vi "String to Array.vi"(0 "string":string, 1 "delimiter (;)":string=";") -> (2 "array":string[](array[string]))   [LabVIEW 2017]
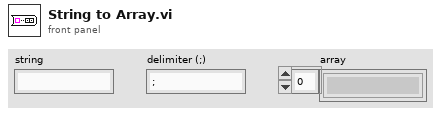
[diagram p1: front panel]
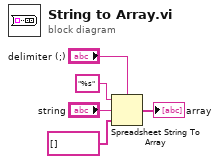
[diagram p0: block diagram]
diagram:
  n1 = Spreadsheet String To Array(delimiter (Tab)="delimiter (;)", format string="%s", spreadsheet string="string", array type (2D Dbl)=string[] [] ("array")) -> (array=→"array":string[])
